vi "PH_Beamline_Common.set Lens in Shotmode Condition.vi"(2 "CtlRef":refnum<vi>, 3 "State":T1 items=["unknown", "Position I", "Position II", "Position III", "Position IV", "moving"], 4 "no link":bool, 5 "error in (no error)":errorcluster) -> (19 "error out":errorcluster)   [LabVIEW 2014, in "PH_Beamline_Common.lvlib"]
uses:
  PH_Beamline_Common.lvlib
  PH_4_Pos_Selector/PH_4_Pos_Selector.Position Selector.ctl
  PH_Common/PH_Common.lvlib
  PH_4_Pos_Selector/PH_4_Pos_Selector.lvlib
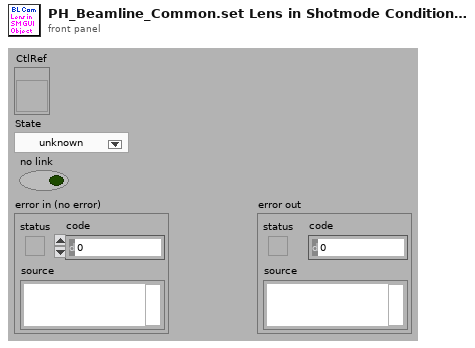
[diagram p1: front panel]
types:
  T1 = typedef "PH_4_Pos_Selector.lvlib/PH_4_Pos_Selector.Position Selector.ctl" = u16
  T2 = cluster{"left":i16, "top":i16, "right":i16, "bottom":i16}
  T3 = cluster{"Width":u16, "Style":enum32{"Solid", "Dash", "Dot", "DashDot", "DashDotDot"}}
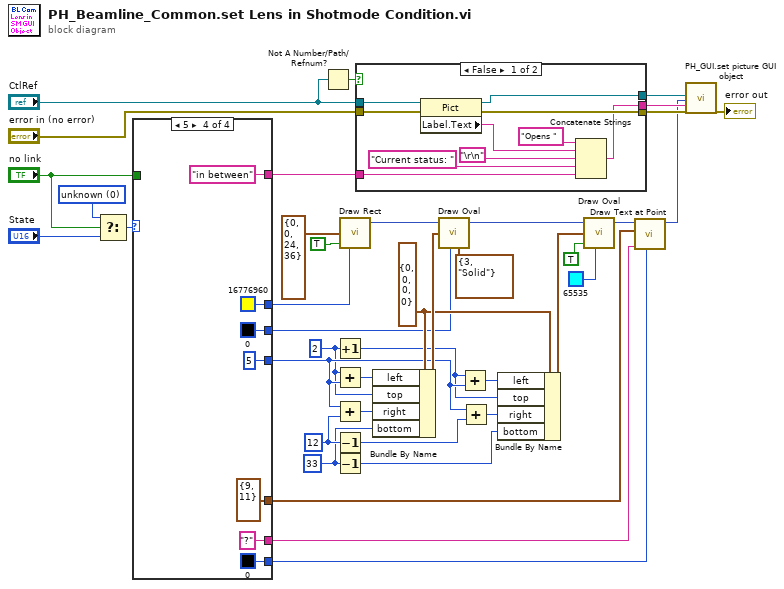
[diagram p0: block diagram]
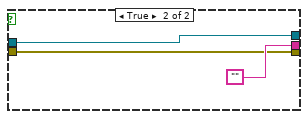
[diagram p2: hidden frame]
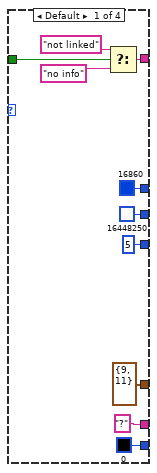
[diagram p3: hidden frame]
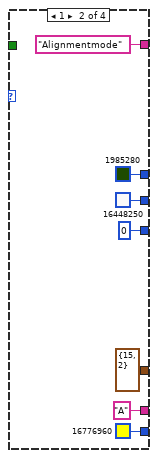
[diagram p4: hidden frame]
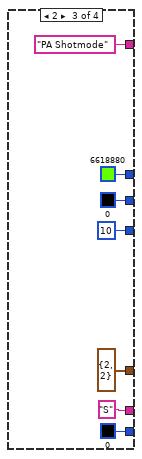
[diagram p5: hidden frame]
diagram:
  w1 = T1 0 items=["unknown", "Position I", "Position II", "Position III", "Position IV", "moving"] ("State")
  w13 = i16 33 ("bottom")
  w11 = i16 2 ("top")
  w15 = i16 12 ("bottom")
  w17 = T2 {"left"=0, "top"=0, "right"=0, "bottom"=0} ("rect")
  n1 = Select(t=w1, s="no link", f="State") -> (s? t:f=w31:T1)
  n2 = case shown="5" w31 {
    tunnel: [u32 16860 u32 1985280 u32 6618880 u32 16776960] -> w34
    tunnel: "no link" -> [w46 _ _ _]
    tunnel: [w47 "Alignmentmode" "PA Shotmode" "in between"] -> w30
    tunnel: [i16 5 ("top") i16 0 ("top") i16 10 ("top") i16 5 ("top")] -> w16
    tunnel: [u32 16448250 u32 16448250 u32 0 u32 0] -> w6
    tunnel: ["?" "A" "S" "?"] -> w7
    tunnel: [u32 0 u32 16776960 u32 0 u32 0] -> w5
    tunnel: [cluster{"x":i16, "y":i16} {"x"=9, "y"=11} ("origin") cluster{"x":i16, "y":i16} {"x"=15, "y"=2} ("origin") cluster{"x":i16, "y":i16} {"x"=2, "y"=2} ("origin") cluster{"x":i16, "y":i16} {"x"=9, "y"=11} ("origin")] -> w4
    frame Default {
      n3 = Select(t="not linked", s=w46, f="no info") -> (s? t:f=w47:string)
    }
    frame 1 {
    }
    frame 2 {
    }
    frame 5 {
    }
  }
  n4 = Not A Number/Path/Refnum?(number/path/refnum="CtlRef") -> (NaN/Path/Refnum?=w2:bool)
  n5 = Increment(x=w11) -> (x+1=w10:i16)
  n6 = Add(x=w11, y=w16) -> (x+y=w20:i16)
  n7 = Add(x=w16, y=w15) -> (x+y=w19:i16)
  n8 = Decrement(x=w15) -> (x-1=w14:i16)
  n9 = Decrement(x=w13) -> (x-1=w12:i16)
  n10 = call <vilib>:"Draw Rect.vi"("rect"=T2 {"left"=0, "top"=0, "right"=24, "bottom"=36}, "fill?(F)"=TRUE, "color(black)"=w34) -> ("new picture"=w23:picture)  [unwired: 6 in]
  n11 = case shown="False" w2 {
    tunnel: "CtlRef" -> [w77 w84]
    tunnel: "error in (no error)" -> [w76 w82]
    tunnel: [w75 w82] -> w32
    tunnel: w30 -> [w74 _]
    tunnel: [w73 ""] -> w29
    tunnel: [w72 w84] -> w3
    frame False {
      n12 = property class="Pict"(reference=w77, error in=w76) -> (reference out=w72:refnum<vi>, error out=w75:errorcluster, "Label.Text"=w80:string)
      n13 = Concatenate Strings("Opens " ("string"), w80, "\r\n", "Current status: " ("string"), w74) -> (w73:string)
    }
    frame True {
    }
  }
  n14 = Bundle By Name(cluster=w17, "left"=w20, "top"=w11, "right"=w19, "bottom"=w13) -> (w18:T2)
  n15 = call <vilib>:"Draw Oval.vi"("picture"=w23, "rect"=w18, "color(black)"=w6, "pen"=T3 {"Width"=3, "Style"=enum."Solid"}) -> ("new picture"=w22:picture)  [unwired: 5 in]
  n16 = Add(x=w10, y=w16) -> (x+y=w28:i16)
  n17 = Add(x=w16, y=w14) -> (x+y=w27:i16)
  n18 = Bundle By Name(cluster=w17, "left"=w28, "top"=w10, "right"=w27, "bottom"=w12) -> (w26:T2)
  n19 = call <vilib>:"Draw Oval.vi"("picture"=w22, "rect"=w26, "fill?(F)"=TRUE, "color(black)"=u32 65535) -> ("new picture"=w9:picture)  [unwired: 5 in]
  n20 = call <vilib>:"Draw Text at Point.vi"("text color(black)"=w5, "text"=w7, "origin"=w4, "picture"=w9) -> ("new picture"=w8:picture)  [unwired: 6 in, 1 out]
  n21 = call "PH_GUI.set picture GUI object.vi"("CtlRef"=w3, "Picture"=w8, "Tip Strip (\"\")"=w29, "error in (no error)"=w32) -> ("error out"=→"error out":errorcluster)  [unwired: 15 in]
